vi "Determine WArning.vi"() -> ()   [LabVIEW 2014]
panel:
  out "Warning?":bool
  out "Warning Text":string
  in  "Min Temp":dbl
  in  "Max Temp":dbl
  in  "Current Temp":dbl
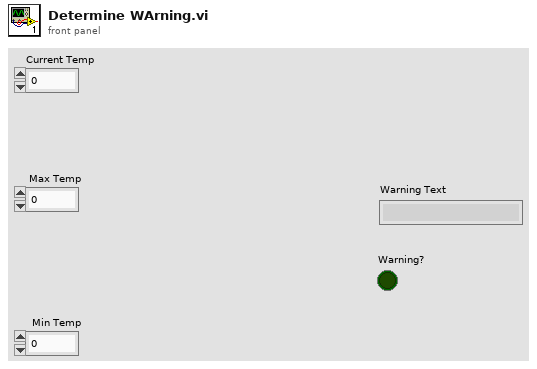
[diagram p1: front panel]
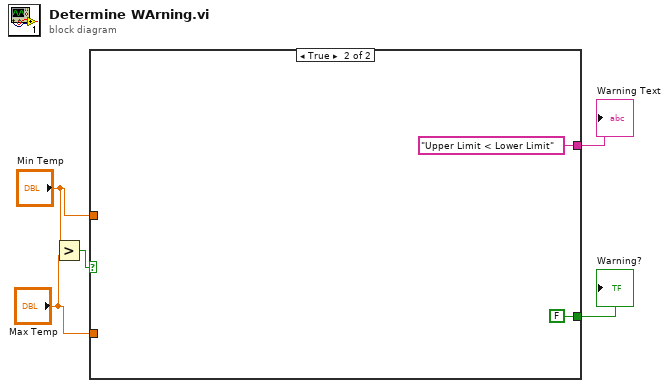
[diagram p0: block diagram]
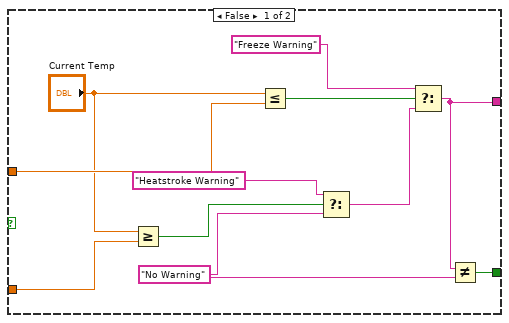
[diagram p2: hidden frame]
diagram:
  n1 = Greater?(x="Min Temp", y="Max Temp") -> (0:w1:bool)
  n2 = case shown="True" w1 {
    tunnel: "Max Temp" -> [w16 _]
    tunnel: "Min Temp" -> [w15 _]
    tunnel: [w8 "Upper Limit < Lower Limit"] -> w5
    tunnel: [w6 FALSE] -> w4
    frame False {
      w7 = "No Warning"
      n3 = Greater Or Equal?(x="Current Temp", y=w16) -> (x >= y?=w13:bool)
      n4 = Less Or Equal?(x="Current Temp", y=w15) -> (x <= y?=w11:bool)
      n5 = Select(t="Heatstroke Warning", s=w13, f=w7) -> (s? t:f=w9:string)
      n6 = Select(t="Freeze Warning", s=w11, f=w9) -> (s? t:f=w8:string)
      n7 = Not Equal?(x=w8, y=w7) -> (x != y?=w6:bool)
    }
    frame True {
    }
  }
  "Warning Text" <- w5
  "Warning?" <- w4
